vi "GlobalVariableTest.vi"() -> ()   [LabVIEW 2020]
panel:
  in  "LeftMotor":dbl
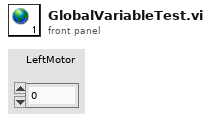
[diagram p1: front panel]
diagram:
